vi "HTML Hierarhy Close.vi"(8 "error in":errorcluster) -> (0 "error out":errorcluster)   [LabVIEW 2014, in "lvprj2html.lvlib"]
uses:
  lvprj2html.lvlib
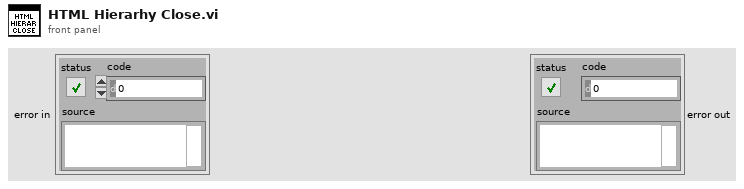
[diagram p1: front panel]
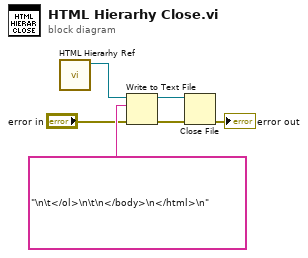
[diagram p0: block diagram]
diagram:
  n1 = call "HTML Hierarhy Ref.vi"() -> ("Byte Stream File out"=w6:refnum<file>)  [unwired: 11 in]
  n2 = Write to Text File(file (use dialog)=w6, text="\n\t</ol>\n\t\n</body>\n</html>\n", error in="error in") -> (refnum out=w5:refnum<file>, error out=w2:errorcluster)  [unwired: 1 in, 1 out]
  n3 = Close File(refnum=w5, error in=w2) -> (error out=→"error out":errorcluster)  [unwired: 1 out]
